vi "Auto Collimation.vi"(8 "error in (no error)":errorcluster, 10 "SN":string, 11 "Fiber Auto Collimation state data in":refnum<class "Fiber Auto Collimation state data.lvclass">) -> (0 "error out":errorcluster caption="error out (no error)", 1 "Cancel Test":bool, 2 "BV Data":T1={"Centroid X[um]"=nan, "Centroid Y[um]"=nan, "PeakResp.[%]"=nan, "Knife Edge X[mm]"=nan, "Knife Edge Y[mm]"=nan, "Circularity"=nan, "Collimation Result"=FALSE} {"PeakResp.[%]" format="%.0g"}, 3 "Fiber Auto Collimation state data out":refnum<class "Fiber Auto Collimation state data.lvclass">, 4 "Stop Position":dbl[unit], 5 "Collimation result":bool)   [LabVIEW 2018]
uses:
  State data/BV Data.ctl
  State data/Fiber Auto Collimation state data.lvclass
  <instrlib>/nLight Instruments/Beam Profiler/Beam Profiler.lvclass
  <instrlib>/nLight Instruments/Motion Controller/Motion Controller.lvclass
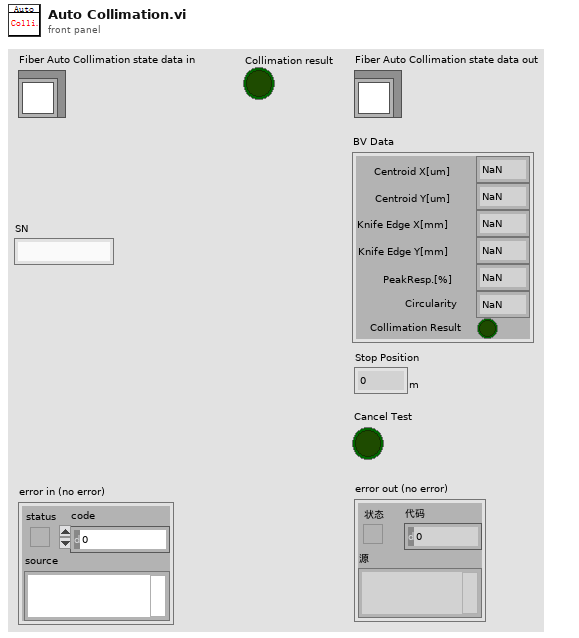
[diagram p1: front panel]
types:
  T1 = typedef "Fiber Auto Collimation state data.lvclass/BV Data.ctl" = cluster{"Centroid X[um]":sgl, "Centroid Y[um]":sgl, "PeakResp.[%]":dbl, "Knife Edge X[mm]":sgl, "Knife Edge Y[mm]":sgl, "Circularity":sgl, "Collimation Result":bool}
  T2 = typedef "Test Parameters.ctl" = cluster{"Start position":dbl, "Peak Resp_min":dbl, "Circularity_min":dbl, "Beam Size Target":dbl, "Beam Size Percentage ":dbl, "Collimation Steps Data Path":string, "Collimation Data Path":string, "Defect detection Image Path":string, "Save Collimation Steps Data Enable":bool, "Defect detection Enable":bool, "Stop position":dbl}
  T3 = typedef "Beam Profiler.lvclass/Beam profiler XY distance value pair.ctl" = cluster{"X":dbl[unit], "Y":dbl[unit]}
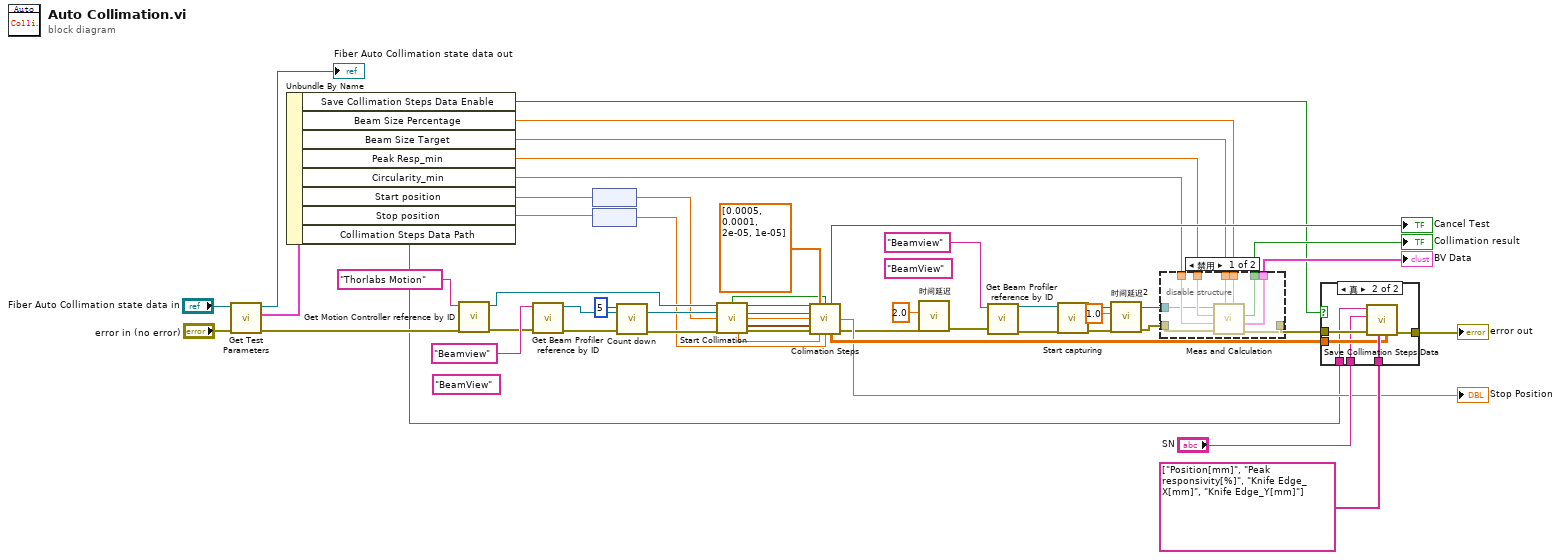
[diagram p0: block diagram]
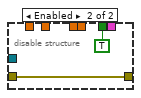
[diagram p2: hidden frame]
diagram:
  (unwired) "BeamView"
  (unwired) "BeamView"
  n1 = call "Get Test Parameters.vi"("error in (no error)"="error in (no error)", "Fiber Auto Collimation state data in"="Fiber Auto Collimation state data in") -> ("error out"=w30:errorcluster, "TestParameters"=w28:T2, "Fiber Auto Collimation state data out"=→"Fiber Auto Collimation state data out":refnum<class "Fiber Auto Collimation state data.lvclass">)  [unwired: 7 in]
  n2 = Unbundle By Name(w28) -> ("Save Collimation Steps Data Enable"=w18:bool, "Beam Size Percentage"=w25:dbl, "Beam Size Target"=w24:dbl, "Peak Resp_min"=w23:dbl, "Circularity_min"=w22:dbl, "Start position"=w27:dbl, "Stop position"=w7:dbl, "Collimation Steps Data Path"=w8:string)
  n3 = call <instrlib>:"Get Motion Controller reference by ID.vi"("error in (no error)"=w30, "Identifier"="Thorlabs Motion") -> ("error out"=w4:errorcluster, "Motion Controller out"=w48:refnum<class "Motion Controller.lvclass">)  [unwired: 8 in]
  n4 = call <instrlib>:"Get Beam Profiler reference by ID.vi"("error in (no error)"=w4, "Identifier"="Beamview") -> ("error out"=w3:errorcluster, "Beam Profiler out"=w47:refnum<class "Beam Profiler.lvclass">)  [unwired: 8 in]
  n5 = node(w27) -> (w26:dbl[unit])
  n6 = node(w7) -> (w6:dbl[unit])
  n7 = call "Count down.vi"("error in (no error)"=w3, "Time"=5) -> ("error out"=w20:errorcluster)  [unwired: 9 in]
  n8 = call "Start Collimation.vi"("Motion Controller in"=w48, "Beam Profiler in"=w47, "Start position"=w26, "error in (no error)"=w20) -> ("Cancel Test"=w37:bool, "Motion Controller out"=w46:refnum<class "Motion Controller.lvclass">, "Beam Profiler out"=w45:refnum<class "Beam Profiler.lvclass">, "Peak responsivity [%,0-100]"=w44:dbl, "Knife Edge"=w43:T3, "Stop position"=w41:dbl[unit], "error out"=w42:errorcluster)  [unwired: 5 in]
  n9 = call "Colimation Steps.vi"("Motion Controller in"=w46, "Steps"=dbl[unit][] [0.0005, 0.0001, 2e-05, 1e-05], "Cancel?"=w37, "Beam Profiler in"=w45, "Peak responsivity [%,0-100]"=w44, "Knife Edge in"=w43, "Error in"=w42, "Start Position"=w41, "Stop Collimation Position"=w6) -> ("Cancel Test"=→"Cancel Test":bool, "Stop Position"=→"Stop Position":dbl[unit], "Steps data"=w32:dbl[][], "Error out"=w1:errorcluster)  [unwired: 1 in, 2 out]
  n10 = call "时间延迟"("error in (no error)"=w1, "Delay Time (s)"=2.0) -> ("error out"=w17:errorcluster)  [unwired: 9 in]
  n11 = call <instrlib>:"Get Beam Profiler reference by ID.vi"("error in (no error)"=w17, "Identifier"="Beamview") -> ("error out"=w16:errorcluster, "Beam Profiler out"=w14:refnum<class "Beam Profiler.lvclass">)  [unwired: 8 in]
  n12 = call-dynamic "Start capturing.vi"("error in (no error)"=w16, "Beam Profiler in"=w14) -> ("error out"=w11:errorcluster, "Beam Profiler out"=w15:refnum<class "Beam Profiler.lvclass">)  [unwired: 8 in]
  n13 = call "时间延迟2"("error in (no error)"=w11, "Delay Time (s)"=1.0) -> ("error out"=w10:errorcluster)  [unwired: 9 in]
  n14 = disable-structure shown="禁用" {
    disable-tunnel: [w59 TRUE ("Collimation result")] -> w40
    disable-tunnel: [w58 _] -> w39
    disable-tunnel: [w57 w61] -> w35
    disable-tunnel: w25 -> [w56 _]
    disable-tunnel: w24 -> [w55 _]
    disable-tunnel: w23 -> [w54 _]
    disable-tunnel: w22 -> [w53 _]
    disable-tunnel: w10 -> [w52 w61]
    disable-tunnel: w15 -> [w51 _]
    frame Disabled {
      n15 = call "Meas and Calculation.vi"("Beam Size Percentage"=w56, "Beam Size Target"=w55, "error in (no error)"=w52, "Circularity_min"=w53, "Peak Resp_min"=w54, "Beam Profiler in"=w51) -> ("error out"=w57:errorcluster, "BV Data"=w58:T1, "Collimation result"=w59:bool)  [unwired: 2 in, 1 out]
    }
    frame Enabled {
    }
  }
  "Collimation result" <- w40
  "BV Data" <- w39
  n16 = case shown="真" w18 {
    tunnel: w35 -> [w62 w68]
    tunnel: [w62 w67] -> w34
    tunnel: string[] ["Position[mm]", "Peak responsivity[%]", "Knife Edge_X[mm]", "Knife Edge_Y[mm]"] ("Item") -> [_ w66]
    tunnel: w32 -> [_ w65]
    tunnel: "SN" -> [_ w64]
    tunnel: w8 -> [_ w63]
    frame False {
    }
    frame True {
      n17 = call "Save Collimation Steps Data.vi"("Data"=w65, "Item"=w66, "Error In"=w68, "SN"=w64, "路径"=w63) -> ("error out"=w67:errorcluster)  [unwired: 6 in]
    }
  }
  "error out" <- w34
